vi "Experiment 16.vi"() -> ()   [LabVIEW 2026]
doc: "Experiment 16\nThis experiment is like Experiment 13 but uses while loops instead of for loops."
uses:
  <vilib>/AdvancedString/1D String Array to Delimited String (string).vi
  <vilib>/Analysis/baseanly.llb/Mean (DBL).vi
  <vilib>/Analysis/NI_AALBase.lvlib
panel:
  out "No. Of Iterations As Block Of Text (easy to copy into Excel)":string
  out "No. Of Iterations Executed - Loop 4":i32
  out "Output - Loop 4":dbl[](array[numeric]) format="%.3f"
  out "No. Of Iterations Executed - Loop 3":i32
  out "Output - Loop 3":dbl[](array[numeric]) format="%.3f"
  out "Avg. No. Of Iterations Executed - All Loops":dbl format="%.1f"
  out "No. Of Iterations Executed - Loop 2":i32
  out "Output - Loop 2":dbl[](array[numeric]) format="%.3f"
  out "No. Of Iterations Executed - Loop 1":i32
  out "Output - Loop 1":dbl[](array[numeric]) format="%.3f"
  out "Stop VI?":bool
  # "Experiment 16"
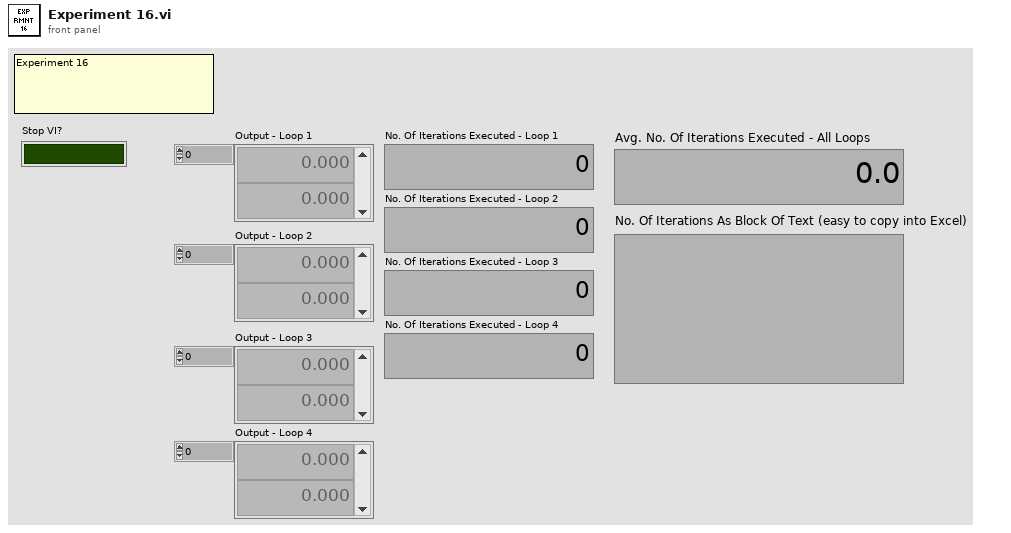
[diagram p1: front panel]
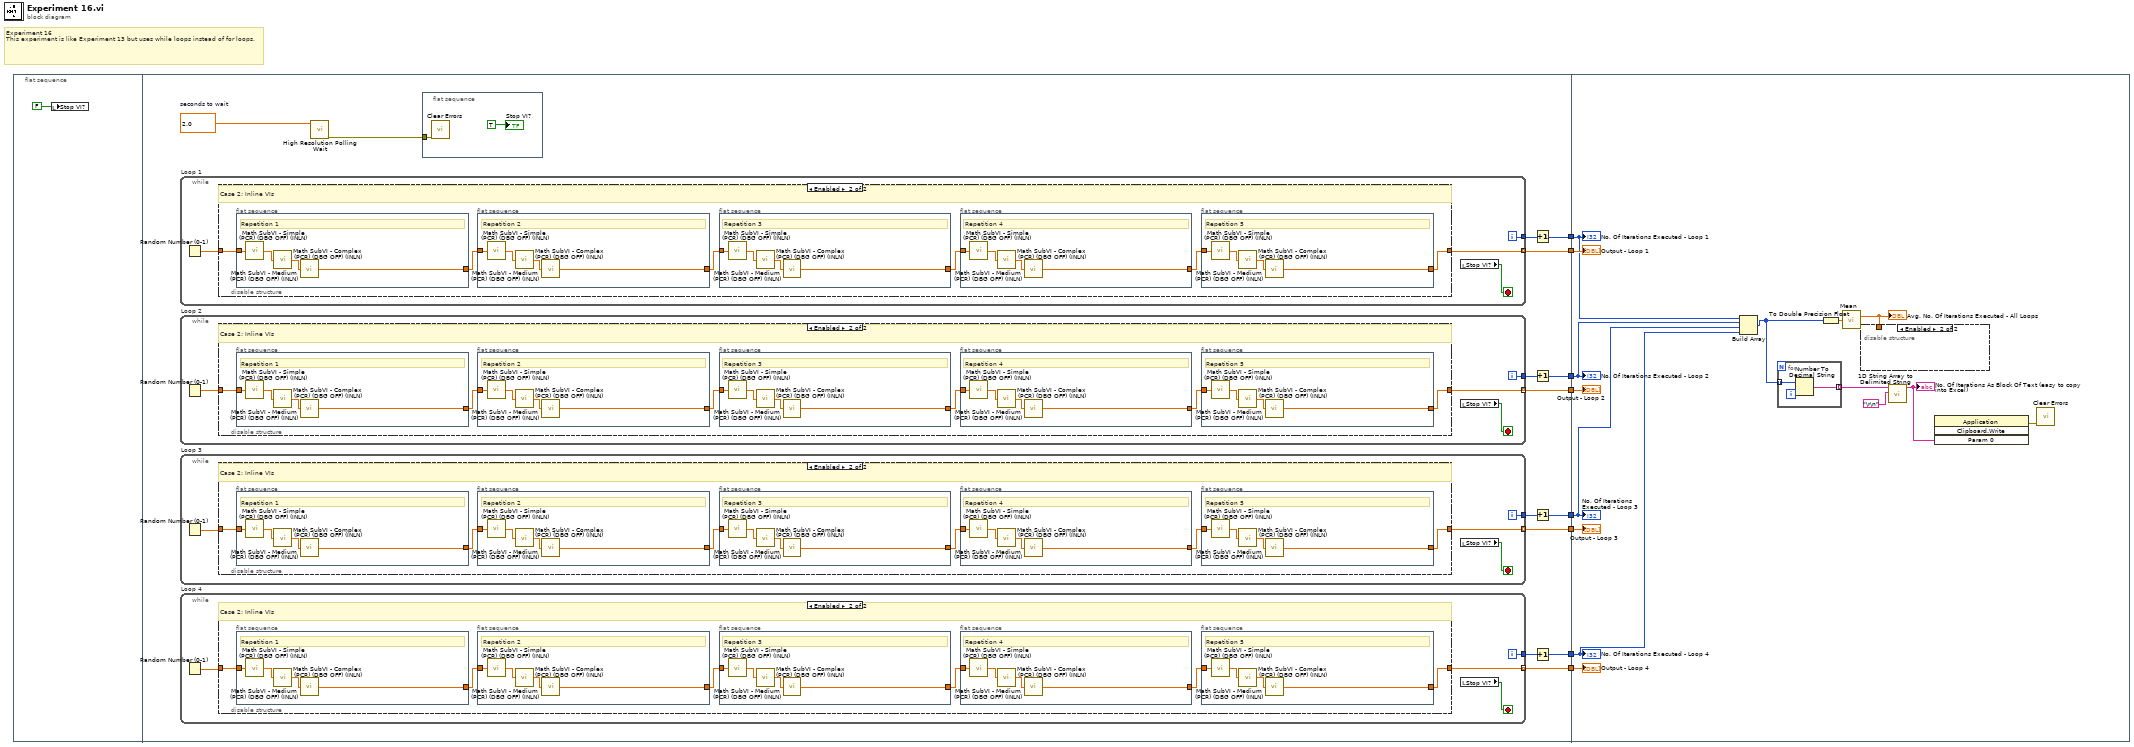
[diagram p0: block diagram]
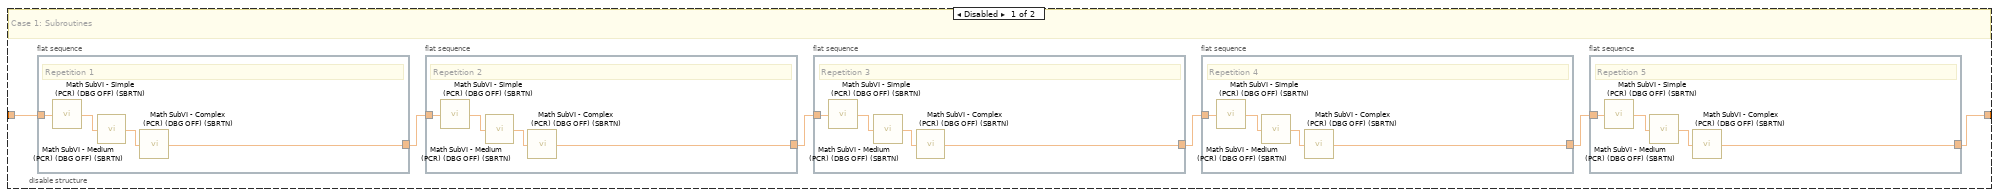
[diagram p2: hidden frame]
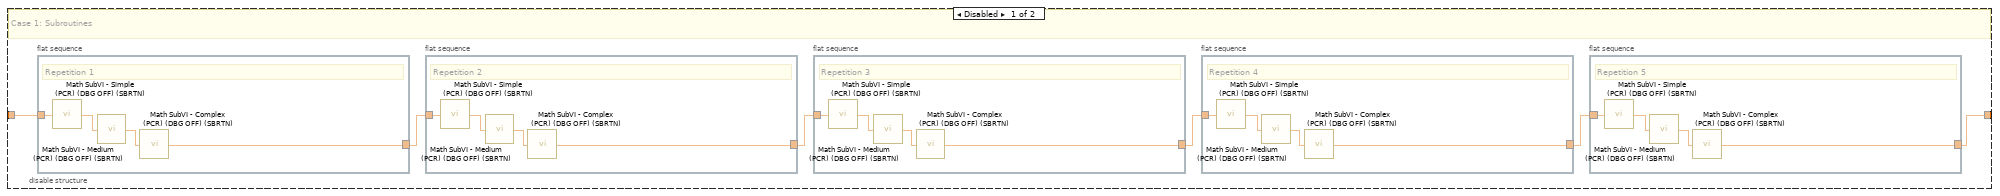
[diagram p3: hidden frame]
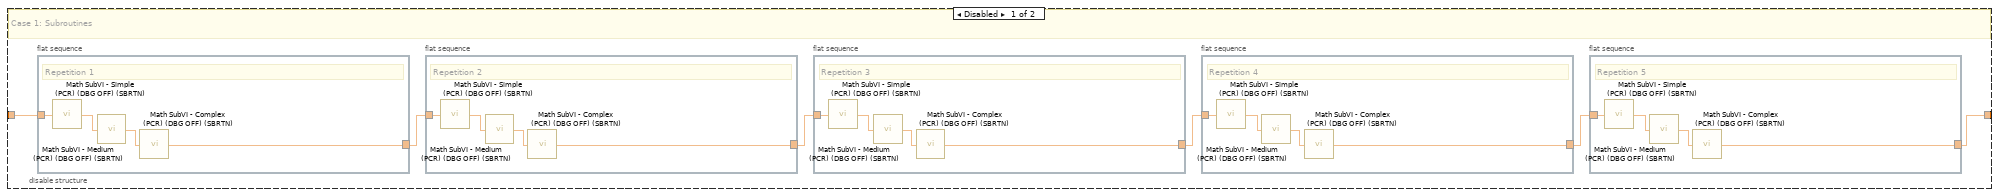
[diagram p4: hidden frame]
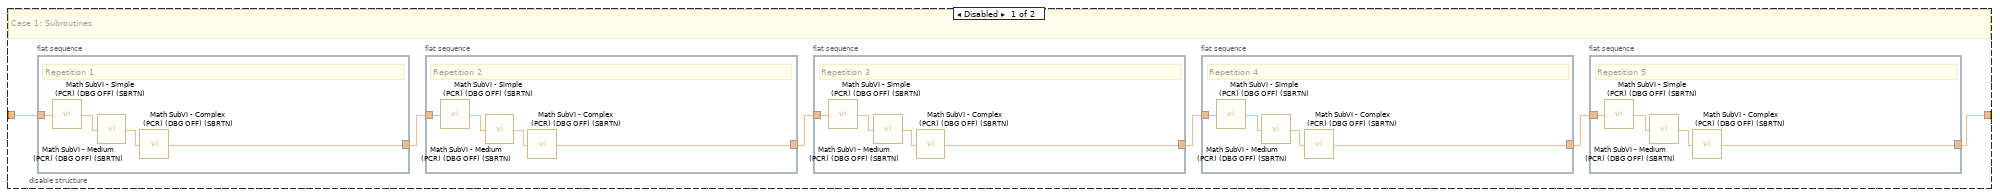
[diagram p5: hidden frame]
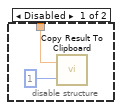
[diagram p6: hidden frame]
diagram:
  # "Experiment 16\nThis experiment is like Experiment 13 but uses while loops instead of for loops."
  n1 = flat-sequence {
    tunnel: [w21] -> w8
    tunnel: [w19] -> w7
    tunnel: [w18] -> w6
    tunnel: [w15] -> w5
    tunnel: [w17] -> w4
    tunnel: [w13] -> w3
    tunnel: [w11] -> w2
    tunnel: [w16] -> w1
    tunnel: w8 -> [w264]
    tunnel: w7 -> [w262]
    tunnel: w6 -> [w261]
    tunnel: w5 -> [w263]
    tunnel: w4 -> [w257]
    tunnel: w3 -> [w259]
    tunnel: w2 -> [w258]
    tunnel: w1 -> [w256]
    frame #0 {
      n2 = local write "Stop VI?"(FALSE) -> ()
    }
    frame #1 {
      w23 = 2.0  # seconds to wait
      n3 = while "Loop 1" {
        tunnel: [w193] -> w21 mode=indexing
        tunnel: [w194] -> w20
        i -> [w194]
        stop <- w195 stop-if-true
        n4 = Random Number (0-1)() -> (number: 0 to 1=w192:dbl)
        n5 = disable-structure shown="Enabled" {
          disable-tunnel: w192 -> [w201 w227]
          disable-tunnel: [w200 w222] -> w193
          frame Disabled {
            # "Case 1: Subroutines"
            n6 = flat-sequence {
              tunnel: w201 -> [w221]
              tunnel: [w218] -> w196
              frame #0 {
                # "Repetition 1"
                n7 = call "Math SubVI - Simple (PCR) (DBG OFF) (SBRTN).vi"("Input"=w221) -> ("Output"=w219:dbl)
                n8 = call "Math SubVI - Medium (PCR) (DBG OFF) (SBRTN).vi"("Input"=w219) -> ("Output"=w220:dbl)
                n9 = call "Math SubVI - Complex (PCR) (DBG OFF) (SBRTN).vi"("Input"=w220) -> ("Output"=w218:dbl)
              }
            }
            n10 = flat-sequence {
              tunnel: w196 -> [w217]
              tunnel: [w214] -> w199
              frame #0 {
                # "Repetition 2"
                n11 = call "Math SubVI - Simple (PCR) (DBG OFF) (SBRTN).vi"("Input"=w217) -> ("Output"=w215:dbl)
                n12 = call "Math SubVI - Medium (PCR) (DBG OFF) (SBRTN).vi"("Input"=w215) -> ("Output"=w216:dbl)
                n13 = call "Math SubVI - Complex (PCR) (DBG OFF) (SBRTN).vi"("Input"=w216) -> ("Output"=w214:dbl)
              }
            }
            n14 = flat-sequence {
              tunnel: w199 -> [w213]
              tunnel: [w210] -> w198
              frame #0 {
                # "Repetition 3"
                n15 = call "Math SubVI - Simple (PCR) (DBG OFF) (SBRTN).vi"("Input"=w213) -> ("Output"=w211:dbl)
                n16 = call "Math SubVI - Medium (PCR) (DBG OFF) (SBRTN).vi"("Input"=w211) -> ("Output"=w212:dbl)
                n17 = call "Math SubVI - Complex (PCR) (DBG OFF) (SBRTN).vi"("Input"=w212) -> ("Output"=w210:dbl)
              }
            }
            n18 = flat-sequence {
              tunnel: w198 -> [w209]
              tunnel: [w206] -> w197
              frame #0 {
                # "Repetition 4"
                n19 = call "Math SubVI - Simple (PCR) (DBG OFF) (SBRTN).vi"("Input"=w209) -> ("Output"=w207:dbl)
                n20 = call "Math SubVI - Medium (PCR) (DBG OFF) (SBRTN).vi"("Input"=w207) -> ("Output"=w208:dbl)
                n21 = call "Math SubVI - Complex (PCR) (DBG OFF) (SBRTN).vi"("Input"=w208) -> ("Output"=w206:dbl)
              }
            }
            n22 = flat-sequence {
              tunnel: w197 -> [w205]
              tunnel: [w202] -> w200
              frame #0 {
                # "Repetition 5"
                n23 = call "Math SubVI - Simple (PCR) (DBG OFF) (SBRTN).vi"("Input"=w205) -> ("Output"=w203:dbl)
                n24 = call "Math SubVI - Medium (PCR) (DBG OFF) (SBRTN).vi"("Input"=w203) -> ("Output"=w204:dbl)
                n25 = call "Math SubVI - Complex (PCR) (DBG OFF) (SBRTN).vi"("Input"=w204) -> ("Output"=w202:dbl)
              }
            }
          }
          frame Enabled {
            # "Case 2: Inline VIs"
            n26 = flat-sequence {
              tunnel: w227 -> [w247]
              tunnel: [w244] -> w226
              frame #0 {
                # "Repetition 1"
                n27 = call "Math SubVI - Simple (PCR) (DBG OFF) (INLN).vi"("Input"=w247) -> ("Output"=w245:dbl)
                n28 = call "Math SubVI - Medium (PCR) (DBG OFF) (INLN).vi"("Input"=w245) -> ("Output"=w246:dbl)
                n29 = call "Math SubVI - Complex (PCR) (DBG OFF) (INLN).vi"("Input"=w246) -> ("Output"=w244:dbl)
              }
            }
            n30 = flat-sequence {
              tunnel: w226 -> [w243]
              tunnel: [w240] -> w225
              frame #0 {
                # "Repetition 2"
                n31 = call "Math SubVI - Simple (PCR) (DBG OFF) (INLN).vi"("Input"=w243) -> ("Output"=w241:dbl)
                n32 = call "Math SubVI - Medium (PCR) (DBG OFF) (INLN).vi"("Input"=w241) -> ("Output"=w242:dbl)
                n33 = call "Math SubVI - Complex (PCR) (DBG OFF) (INLN).vi"("Input"=w242) -> ("Output"=w240:dbl)
              }
            }
            n34 = flat-sequence {
              tunnel: w225 -> [w239]
              tunnel: [w236] -> w224
              frame #0 {
                # "Repetition 3"
                n35 = call "Math SubVI - Simple (PCR) (DBG OFF) (INLN).vi"("Input"=w239) -> ("Output"=w237:dbl)
                n36 = call "Math SubVI - Medium (PCR) (DBG OFF) (INLN).vi"("Input"=w237) -> ("Output"=w238:dbl)
                n37 = call "Math SubVI - Complex (PCR) (DBG OFF) (INLN).vi"("Input"=w238) -> ("Output"=w236:dbl)
              }
            }
            n38 = flat-sequence {
              tunnel: w224 -> [w235]
              tunnel: [w232] -> w223
              frame #0 {
                # "Repetition 4"
                n39 = call "Math SubVI - Simple (PCR) (DBG OFF) (INLN).vi"("Input"=w235) -> ("Output"=w233:dbl)
                n40 = call "Math SubVI - Medium (PCR) (DBG OFF) (INLN).vi"("Input"=w233) -> ("Output"=w234:dbl)
                n41 = call "Math SubVI - Complex (PCR) (DBG OFF) (INLN).vi"("Input"=w234) -> ("Output"=w232:dbl)
              }
            }
            n42 = flat-sequence {
              tunnel: w223 -> [w231]
              tunnel: [w228] -> w222
              frame #0 {
                # "Repetition 5"
                n43 = call "Math SubVI - Simple (PCR) (DBG OFF) (INLN).vi"("Input"=w231) -> ("Output"=w229:dbl)
                n44 = call "Math SubVI - Medium (PCR) (DBG OFF) (INLN).vi"("Input"=w229) -> ("Output"=w230:dbl)
                n45 = call "Math SubVI - Complex (PCR) (DBG OFF) (INLN).vi"("Input"=w230) -> ("Output"=w228:dbl)
              }
            }
          }
        }
        n46 = local read "Stop VI?"() -> (w195:bool)
      }
      n47 = while "Loop 2" {
        tunnel: [w137] -> w15 mode=indexing
        tunnel: [w138] -> w14
        i -> [w138]
        stop <- w139 stop-if-true
        n48 = Random Number (0-1)() -> (number: 0 to 1=w136:dbl)
        n49 = disable-structure shown="Enabled" {
          disable-tunnel: w136 -> [w145 w171]
          disable-tunnel: [w144 w166] -> w137
          frame Disabled {
            # "Case 1: Subroutines"
            n50 = flat-sequence {
              tunnel: w145 -> [w165]
              tunnel: [w162] -> w140
              frame #0 {
                # "Repetition 1"
                n51 = call "Math SubVI - Simple (PCR) (DBG OFF) (SBRTN).vi"("Input"=w165) -> ("Output"=w163:dbl)
                n52 = call "Math SubVI - Medium (PCR) (DBG OFF) (SBRTN).vi"("Input"=w163) -> ("Output"=w164:dbl)
                n53 = call "Math SubVI - Complex (PCR) (DBG OFF) (SBRTN).vi"("Input"=w164) -> ("Output"=w162:dbl)
              }
            }
            n54 = flat-sequence {
              tunnel: w140 -> [w161]
              tunnel: [w158] -> w143
              frame #0 {
                # "Repetition 2"
                n55 = call "Math SubVI - Simple (PCR) (DBG OFF) (SBRTN).vi"("Input"=w161) -> ("Output"=w159:dbl)
                n56 = call "Math SubVI - Medium (PCR) (DBG OFF) (SBRTN).vi"("Input"=w159) -> ("Output"=w160:dbl)
                n57 = call "Math SubVI - Complex (PCR) (DBG OFF) (SBRTN).vi"("Input"=w160) -> ("Output"=w158:dbl)
              }
            }
            n58 = flat-sequence {
              tunnel: w143 -> [w157]
              tunnel: [w154] -> w142
              frame #0 {
                # "Repetition 3"
                n59 = call "Math SubVI - Simple (PCR) (DBG OFF) (SBRTN).vi"("Input"=w157) -> ("Output"=w155:dbl)
                n60 = call "Math SubVI - Medium (PCR) (DBG OFF) (SBRTN).vi"("Input"=w155) -> ("Output"=w156:dbl)
                n61 = call "Math SubVI - Complex (PCR) (DBG OFF) (SBRTN).vi"("Input"=w156) -> ("Output"=w154:dbl)
              }
            }
            n62 = flat-sequence {
              tunnel: w142 -> [w153]
              tunnel: [w150] -> w141
              frame #0 {
                # "Repetition 4"
                n63 = call "Math SubVI - Simple (PCR) (DBG OFF) (SBRTN).vi"("Input"=w153) -> ("Output"=w151:dbl)
                n64 = call "Math SubVI - Medium (PCR) (DBG OFF) (SBRTN).vi"("Input"=w151) -> ("Output"=w152:dbl)
                n65 = call "Math SubVI - Complex (PCR) (DBG OFF) (SBRTN).vi"("Input"=w152) -> ("Output"=w150:dbl)
              }
            }
            n66 = flat-sequence {
              tunnel: w141 -> [w149]
              tunnel: [w146] -> w144
              frame #0 {
                # "Repetition 5"
                n67 = call "Math SubVI - Simple (PCR) (DBG OFF) (SBRTN).vi"("Input"=w149) -> ("Output"=w147:dbl)
                n68 = call "Math SubVI - Medium (PCR) (DBG OFF) (SBRTN).vi"("Input"=w147) -> ("Output"=w148:dbl)
                n69 = call "Math SubVI - Complex (PCR) (DBG OFF) (SBRTN).vi"("Input"=w148) -> ("Output"=w146:dbl)
              }
            }
          }
          frame Enabled {
            # "Case 2: Inline VIs"
            n70 = flat-sequence {
              tunnel: w171 -> [w191]
              tunnel: [w188] -> w170
              frame #0 {
                # "Repetition 1"
                n71 = call "Math SubVI - Simple (PCR) (DBG OFF) (INLN).vi"("Input"=w191) -> ("Output"=w189:dbl)
                n72 = call "Math SubVI - Medium (PCR) (DBG OFF) (INLN).vi"("Input"=w189) -> ("Output"=w190:dbl)
                n73 = call "Math SubVI - Complex (PCR) (DBG OFF) (INLN).vi"("Input"=w190) -> ("Output"=w188:dbl)
              }
            }
            n74 = flat-sequence {
              tunnel: w170 -> [w187]
              tunnel: [w184] -> w169
              frame #0 {
                # "Repetition 2"
                n75 = call "Math SubVI - Simple (PCR) (DBG OFF) (INLN).vi"("Input"=w187) -> ("Output"=w185:dbl)
                n76 = call "Math SubVI - Medium (PCR) (DBG OFF) (INLN).vi"("Input"=w185) -> ("Output"=w186:dbl)
                n77 = call "Math SubVI - Complex (PCR) (DBG OFF) (INLN).vi"("Input"=w186) -> ("Output"=w184:dbl)
              }
            }
            n78 = flat-sequence {
              tunnel: w169 -> [w183]
              tunnel: [w180] -> w168
              frame #0 {
                # "Repetition 3"
                n79 = call "Math SubVI - Simple (PCR) (DBG OFF) (INLN).vi"("Input"=w183) -> ("Output"=w181:dbl)
                n80 = call "Math SubVI - Medium (PCR) (DBG OFF) (INLN).vi"("Input"=w181) -> ("Output"=w182:dbl)
                n81 = call "Math SubVI - Complex (PCR) (DBG OFF) (INLN).vi"("Input"=w182) -> ("Output"=w180:dbl)
              }
            }
            n82 = flat-sequence {
              tunnel: w168 -> [w179]
              tunnel: [w176] -> w167
              frame #0 {
                # "Repetition 4"
                n83 = call "Math SubVI - Simple (PCR) (DBG OFF) (INLN).vi"("Input"=w179) -> ("Output"=w177:dbl)
                n84 = call "Math SubVI - Medium (PCR) (DBG OFF) (INLN).vi"("Input"=w177) -> ("Output"=w178:dbl)
                n85 = call "Math SubVI - Complex (PCR) (DBG OFF) (INLN).vi"("Input"=w178) -> ("Output"=w176:dbl)
              }
            }
            n86 = flat-sequence {
              tunnel: w167 -> [w175]
              tunnel: [w172] -> w166
              frame #0 {
                # "Repetition 5"
                n87 = call "Math SubVI - Simple (PCR) (DBG OFF) (INLN).vi"("Input"=w175) -> ("Output"=w173:dbl)
                n88 = call "Math SubVI - Medium (PCR) (DBG OFF) (INLN).vi"("Input"=w173) -> ("Output"=w174:dbl)
                n89 = call "Math SubVI - Complex (PCR) (DBG OFF) (INLN).vi"("Input"=w174) -> ("Output"=w172:dbl)
              }
            }
          }
        }
        n90 = local read "Stop VI?"() -> (w139:bool)
      }
      n91 = while "Loop 3" {
        tunnel: [w81] -> w13 mode=indexing
        tunnel: [w82] -> w12
        i -> [w82]
        stop <- w83 stop-if-true
        n92 = Random Number (0-1)() -> (number: 0 to 1=w80:dbl)
        n93 = disable-structure shown="Enabled" {
          disable-tunnel: w80 -> [w89 w115]
          disable-tunnel: [w88 w110] -> w81
          frame Disabled {
            # "Case 1: Subroutines"
            n94 = flat-sequence {
              tunnel: w89 -> [w109]
              tunnel: [w106] -> w84
              frame #0 {
                # "Repetition 1"
                n95 = call "Math SubVI - Simple (PCR) (DBG OFF) (SBRTN).vi"("Input"=w109) -> ("Output"=w107:dbl)
                n96 = call "Math SubVI - Medium (PCR) (DBG OFF) (SBRTN).vi"("Input"=w107) -> ("Output"=w108:dbl)
                n97 = call "Math SubVI - Complex (PCR) (DBG OFF) (SBRTN).vi"("Input"=w108) -> ("Output"=w106:dbl)
              }
            }
            n98 = flat-sequence {
              tunnel: w84 -> [w105]
              tunnel: [w102] -> w87
              frame #0 {
                # "Repetition 2"
                n99 = call "Math SubVI - Simple (PCR) (DBG OFF) (SBRTN).vi"("Input"=w105) -> ("Output"=w103:dbl)
                n100 = call "Math SubVI - Medium (PCR) (DBG OFF) (SBRTN).vi"("Input"=w103) -> ("Output"=w104:dbl)
                n101 = call "Math SubVI - Complex (PCR) (DBG OFF) (SBRTN).vi"("Input"=w104) -> ("Output"=w102:dbl)
              }
            }
            n102 = flat-sequence {
              tunnel: w87 -> [w101]
              tunnel: [w98] -> w86
              frame #0 {
                # "Repetition 3"
                n103 = call "Math SubVI - Simple (PCR) (DBG OFF) (SBRTN).vi"("Input"=w101) -> ("Output"=w99:dbl)
                n104 = call "Math SubVI - Medium (PCR) (DBG OFF) (SBRTN).vi"("Input"=w99) -> ("Output"=w100:dbl)
                n105 = call "Math SubVI - Complex (PCR) (DBG OFF) (SBRTN).vi"("Input"=w100) -> ("Output"=w98:dbl)
              }
            }
            n106 = flat-sequence {
              tunnel: w86 -> [w97]
              tunnel: [w94] -> w85
              frame #0 {
                # "Repetition 4"
                n107 = call "Math SubVI - Simple (PCR) (DBG OFF) (SBRTN).vi"("Input"=w97) -> ("Output"=w95:dbl)
                n108 = call "Math SubVI - Medium (PCR) (DBG OFF) (SBRTN).vi"("Input"=w95) -> ("Output"=w96:dbl)
                n109 = call "Math SubVI - Complex (PCR) (DBG OFF) (SBRTN).vi"("Input"=w96) -> ("Output"=w94:dbl)
              }
            }
            n110 = flat-sequence {
              tunnel: w85 -> [w93]
              tunnel: [w90] -> w88
              frame #0 {
                # "Repetition 5"
                n111 = call "Math SubVI - Simple (PCR) (DBG OFF) (SBRTN).vi"("Input"=w93) -> ("Output"=w91:dbl)
                n112 = call "Math SubVI - Medium (PCR) (DBG OFF) (SBRTN).vi"("Input"=w91) -> ("Output"=w92:dbl)
                n113 = call "Math SubVI - Complex (PCR) (DBG OFF) (SBRTN).vi"("Input"=w92) -> ("Output"=w90:dbl)
              }
            }
          }
          frame Enabled {
            # "Case 2: Inline VIs"
            n114 = flat-sequence {
              tunnel: w115 -> [w135]
              tunnel: [w132] -> w114
              frame #0 {
                # "Repetition 1"
                n115 = call "Math SubVI - Simple (PCR) (DBG OFF) (INLN).vi"("Input"=w135) -> ("Output"=w133:dbl)
                n116 = call "Math SubVI - Medium (PCR) (DBG OFF) (INLN).vi"("Input"=w133) -> ("Output"=w134:dbl)
                n117 = call "Math SubVI - Complex (PCR) (DBG OFF) (INLN).vi"("Input"=w134) -> ("Output"=w132:dbl)
              }
            }
            n118 = flat-sequence {
              tunnel: w114 -> [w131]
              tunnel: [w128] -> w113
              frame #0 {
                # "Repetition 2"
                n119 = call "Math SubVI - Simple (PCR) (DBG OFF) (INLN).vi"("Input"=w131) -> ("Output"=w129:dbl)
                n120 = call "Math SubVI - Medium (PCR) (DBG OFF) (INLN).vi"("Input"=w129) -> ("Output"=w130:dbl)
                n121 = call "Math SubVI - Complex (PCR) (DBG OFF) (INLN).vi"("Input"=w130) -> ("Output"=w128:dbl)
              }
            }
            n122 = flat-sequence {
              tunnel: w113 -> [w127]
              tunnel: [w124] -> w112
              frame #0 {
                # "Repetition 3"
                n123 = call "Math SubVI - Simple (PCR) (DBG OFF) (INLN).vi"("Input"=w127) -> ("Output"=w125:dbl)
                n124 = call "Math SubVI - Medium (PCR) (DBG OFF) (INLN).vi"("Input"=w125) -> ("Output"=w126:dbl)
                n125 = call "Math SubVI - Complex (PCR) (DBG OFF) (INLN).vi"("Input"=w126) -> ("Output"=w124:dbl)
              }
            }
            n126 = flat-sequence {
              tunnel: w112 -> [w123]
              tunnel: [w120] -> w111
              frame #0 {
                # "Repetition 4"
                n127 = call "Math SubVI - Simple (PCR) (DBG OFF) (INLN).vi"("Input"=w123) -> ("Output"=w121:dbl)
                n128 = call "Math SubVI - Medium (PCR) (DBG OFF) (INLN).vi"("Input"=w121) -> ("Output"=w122:dbl)
                n129 = call "Math SubVI - Complex (PCR) (DBG OFF) (INLN).vi"("Input"=w122) -> ("Output"=w120:dbl)
              }
            }
            n130 = flat-sequence {
              tunnel: w111 -> [w119]
              tunnel: [w116] -> w110
              frame #0 {
                # "Repetition 5"
                n131 = call "Math SubVI - Simple (PCR) (DBG OFF) (INLN).vi"("Input"=w119) -> ("Output"=w117:dbl)
                n132 = call "Math SubVI - Medium (PCR) (DBG OFF) (INLN).vi"("Input"=w117) -> ("Output"=w118:dbl)
                n133 = call "Math SubVI - Complex (PCR) (DBG OFF) (INLN).vi"("Input"=w118) -> ("Output"=w116:dbl)
              }
            }
          }
        }
        n134 = local read "Stop VI?"() -> (w83:bool)
      }
      n135 = while "Loop 4" {
        tunnel: [w25] -> w11 mode=indexing
        tunnel: [w26] -> w10
        i -> [w26]
        stop <- w27 stop-if-true
        n136 = Random Number (0-1)() -> (number: 0 to 1=w24:dbl)
        n137 = disable-structure shown="Enabled" {
          disable-tunnel: w24 -> [w33 w59]
          disable-tunnel: [w32 w54] -> w25
          frame Disabled {
            # "Case 1: Subroutines"
            n138 = flat-sequence {
              tunnel: w33 -> [w53]
              tunnel: [w50] -> w28
              frame #0 {
                # "Repetition 1"
                n139 = call "Math SubVI - Simple (PCR) (DBG OFF) (SBRTN).vi"("Input"=w53) -> ("Output"=w51:dbl)
                n140 = call "Math SubVI - Medium (PCR) (DBG OFF) (SBRTN).vi"("Input"=w51) -> ("Output"=w52:dbl)
                n141 = call "Math SubVI - Complex (PCR) (DBG OFF) (SBRTN).vi"("Input"=w52) -> ("Output"=w50:dbl)
              }
            }
            n142 = flat-sequence {
              tunnel: w28 -> [w49]
              tunnel: [w46] -> w31
              frame #0 {
                # "Repetition 2"
                n143 = call "Math SubVI - Simple (PCR) (DBG OFF) (SBRTN).vi"("Input"=w49) -> ("Output"=w47:dbl)
                n144 = call "Math SubVI - Medium (PCR) (DBG OFF) (SBRTN).vi"("Input"=w47) -> ("Output"=w48:dbl)
                n145 = call "Math SubVI - Complex (PCR) (DBG OFF) (SBRTN).vi"("Input"=w48) -> ("Output"=w46:dbl)
              }
            }
            n146 = flat-sequence {
              tunnel: w31 -> [w45]
              tunnel: [w42] -> w30
              frame #0 {
                # "Repetition 3"
                n147 = call "Math SubVI - Simple (PCR) (DBG OFF) (SBRTN).vi"("Input"=w45) -> ("Output"=w43:dbl)
                n148 = call "Math SubVI - Medium (PCR) (DBG OFF) (SBRTN).vi"("Input"=w43) -> ("Output"=w44:dbl)
                n149 = call "Math SubVI - Complex (PCR) (DBG OFF) (SBRTN).vi"("Input"=w44) -> ("Output"=w42:dbl)
              }
            }
            n150 = flat-sequence {
              tunnel: w30 -> [w41]
              tunnel: [w38] -> w29
              frame #0 {
                # "Repetition 4"
                n151 = call "Math SubVI - Simple (PCR) (DBG OFF) (SBRTN).vi"("Input"=w41) -> ("Output"=w39:dbl)
                n152 = call "Math SubVI - Medium (PCR) (DBG OFF) (SBRTN).vi"("Input"=w39) -> ("Output"=w40:dbl)
                n153 = call "Math SubVI - Complex (PCR) (DBG OFF) (SBRTN).vi"("Input"=w40) -> ("Output"=w38:dbl)
              }
            }
            n154 = flat-sequence {
              tunnel: w29 -> [w37]
              tunnel: [w34] -> w32
              frame #0 {
                # "Repetition 5"
                n155 = call "Math SubVI - Simple (PCR) (DBG OFF) (SBRTN).vi"("Input"=w37) -> ("Output"=w35:dbl)
                n156 = call "Math SubVI - Medium (PCR) (DBG OFF) (SBRTN).vi"("Input"=w35) -> ("Output"=w36:dbl)
                n157 = call "Math SubVI - Complex (PCR) (DBG OFF) (SBRTN).vi"("Input"=w36) -> ("Output"=w34:dbl)
              }
            }
          }
          frame Enabled {
            # "Case 2: Inline VIs"
            n158 = flat-sequence {
              tunnel: w59 -> [w79]
              tunnel: [w76] -> w58
              frame #0 {
                # "Repetition 1"
                n159 = call "Math SubVI - Simple (PCR) (DBG OFF) (INLN).vi"("Input"=w79) -> ("Output"=w77:dbl)
                n160 = call "Math SubVI - Medium (PCR) (DBG OFF) (INLN).vi"("Input"=w77) -> ("Output"=w78:dbl)
                n161 = call "Math SubVI - Complex (PCR) (DBG OFF) (INLN).vi"("Input"=w78) -> ("Output"=w76:dbl)
              }
            }
            n162 = flat-sequence {
              tunnel: w58 -> [w75]
              tunnel: [w72] -> w57
              frame #0 {
                # "Repetition 2"
                n163 = call "Math SubVI - Simple (PCR) (DBG OFF) (INLN).vi"("Input"=w75) -> ("Output"=w73:dbl)
                n164 = call "Math SubVI - Medium (PCR) (DBG OFF) (INLN).vi"("Input"=w73) -> ("Output"=w74:dbl)
                n165 = call "Math SubVI - Complex (PCR) (DBG OFF) (INLN).vi"("Input"=w74) -> ("Output"=w72:dbl)
              }
            }
            n166 = flat-sequence {
              tunnel: w57 -> [w71]
              tunnel: [w68] -> w56
              frame #0 {
                # "Repetition 3"
                n167 = call "Math SubVI - Simple (PCR) (DBG OFF) (INLN).vi"("Input"=w71) -> ("Output"=w69:dbl)
                n168 = call "Math SubVI - Medium (PCR) (DBG OFF) (INLN).vi"("Input"=w69) -> ("Output"=w70:dbl)
                n169 = call "Math SubVI - Complex (PCR) (DBG OFF) (INLN).vi"("Input"=w70) -> ("Output"=w68:dbl)
              }
            }
            n170 = flat-sequence {
              tunnel: w56 -> [w67]
              tunnel: [w64] -> w55
              frame #0 {
                # "Repetition 4"
                n171 = call "Math SubVI - Simple (PCR) (DBG OFF) (INLN).vi"("Input"=w67) -> ("Output"=w65:dbl)
                n172 = call "Math SubVI - Medium (PCR) (DBG OFF) (INLN).vi"("Input"=w65) -> ("Output"=w66:dbl)
                n173 = call "Math SubVI - Complex (PCR) (DBG OFF) (INLN).vi"("Input"=w66) -> ("Output"=w64:dbl)
              }
            }
            n174 = flat-sequence {
              tunnel: w55 -> [w63]
              tunnel: [w60] -> w54
              frame #0 {
                # "Repetition 5"
                n175 = call "Math SubVI - Simple (PCR) (DBG OFF) (INLN).vi"("Input"=w63) -> ("Output"=w61:dbl)
                n176 = call "Math SubVI - Medium (PCR) (DBG OFF) (INLN).vi"("Input"=w61) -> ("Output"=w62:dbl)
                n177 = call "Math SubVI - Complex (PCR) (DBG OFF) (INLN).vi"("Input"=w62) -> ("Output"=w60:dbl)
              }
            }
          }
        }
        n178 = local read "Stop VI?"() -> (w27:bool)
      }
      n179 = call <vilib>:"High Resolution Polling Wait.vi"("seconds to wait"=w23) -> ("error out"=w22:errorcluster)  [unwired: 10 in]
      n180 = flat-sequence {
        tunnel: w22 -> [w248]
        frame #0 {
          n181 = call <vilib>:"Clear Errors.vi"("error in (no error)"=w248) -> ()  [unwired: 5 in, 2 out]
          "Stop VI?" <- TRUE
        }
      }
      n182 = Increment(x=w20) -> (x+1=w19:i32)
      n183 = Increment(x=w14) -> (x+1=w18:i32)
      n184 = Increment(x=w12) -> (x+1=w17:i32)
      n185 = Increment(x=w10) -> (x+1=w16:i32)
    }
    frame #2 {
      n186 = Build Array(w262, w261, w257, w256) -> (w254:i32[])
      n187 = for {
        tunnel: w254 -> [w268] mode=indexing
        tunnel: [w267] -> w253 mode=indexing
        n188 = Number To Decimal String(number=w268) -> (decimal integer string=w267:string)  [unwired: 1 in]
      }
      n189 = To Double Precision Float(number=w254) -> (double precision float=w255:dbl[])
      n190 = call-poly <vilib>:"Mean.vi"("X"=w255) -> ("mean"=w260:dbl)  [unwired: 1 out]
      "Avg. No. Of Iterations Executed - All Loops" <- w260
      n191 = disable-structure shown="Enabled" {
        disable-tunnel: w260 -> [w266 _]
        frame Disabled {
          n192 = call "Copy Result To Clipboard.vi"("No. Of Decimal Places (6)"=u32 1, "Input"=w266) -> ()
        }
        frame Enabled {
        }
      }
      n193 = call-poly <vilib>:"1D String Array to Delimited String.vi"("delimiter"="\r\n", "string array"=w253) -> ("delimited string"=w250:string)  [unwired: 9 in]
      "No. Of Iterations As Block Of Text (easy to copy into Excel)" <- w250
      n194 = invoke class="Application" method="Clipboard.Write"("Param 0"=w250) -> (error out=w251:errorcluster)  [unwired: 3 in, 3 out]
      n195 = call <vilib>:"Clear Errors.vi"("error in (no error)"=w251) -> ()  [unwired: 5 in, 2 out]
      "No. Of Iterations Executed - Loop 1" <- w262
      "Output - Loop 1" <- w264
      "No. Of Iterations Executed - Loop 2" <- w261
      "Output - Loop 2" <- w263
      "No. Of Iterations Executed - Loop 3" <- w257
      "Output - Loop 3" <- w259
      "No. Of Iterations Executed - Loop 4" <- w256
      "Output - Loop 4" <- w258
    }
  }
